vi "ReceiveNorification.vi"(8 "error in (no error)":errorcluster, 11 "ForecastDisplay in":refnum<class "Email Notification.lvclass">) -> (0 "error out":errorcluster, 3 "ForecastDisplay Out":refnum<class "Email Notification.lvclass">)   [LabVIEW 2020, in "Email Notification.lvclass"]
uses:
  Email Notification.lvclass
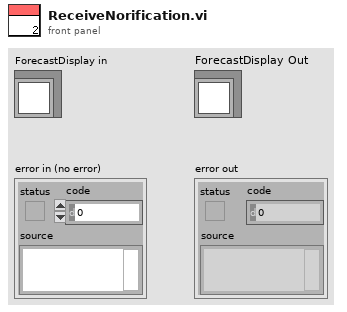
[diagram p1: front panel]
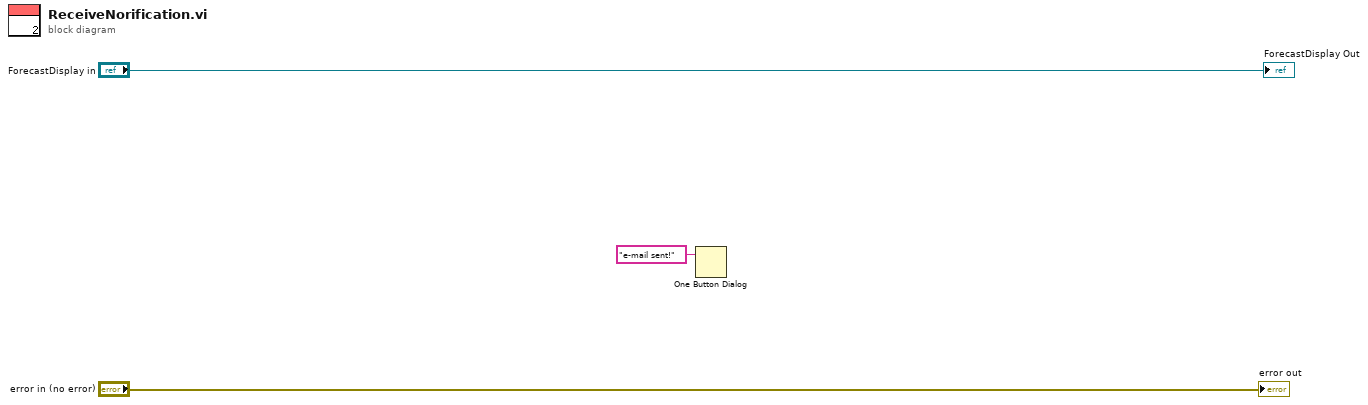
[diagram p0: block diagram]
diagram:
  n1 = One Button Dialog(message="e-mail sent!") -> ()  [unwired: 1 in, 1 out]
  "error out" <- "error in (no error)"
  "ForecastDisplay Out" <- "ForecastDisplay in"
